vi "Read (Single Waveform).vi"(8 "error in (no error)":errorcluster, 9 "Maximum Time (10000ms)":u32=10000, 10 "Channel (0: Channel 1)":u16(ring) items=["Channel 1", "Channel 2", "Channel 3", "Channel 4", "Math", "Reference 1", "Reference 2", "Reference 3", "Reference 4", "D0", "D1", "D2", "D3", "D4", "D5", "D6", "D7", "D8", "D9", "D10", "D11", "D12", "D13", "D14", "D15", "Amplitude", "Frequency", "Phase", "Normal", "Average", "Maximum Peak Hold", "Minimum Peak Hold"], 11 "VISA resource name":refnum<visa-resource-name>) -> (0 "error out":errorcluster, 2 "Waveform Graph":waveform(dbl)(graph), 3 "VISA resource name out":refnum<visa-resource-name>)   [LabVIEW 2013, in "Tektronix DPO MSO 2000 4000 Series.lvlib"]
doc: "Initiates an acquisition on all channels that you enabled with the Configure Channel VI. This VI waits for the acquisition to complete and returns the waveform for the <B> Channel</B> you specify. The <B>Timeout</B> control specifies the maximum time to wait for operation complete in milliseconds. If the oscilloscope does not complete the acquisition within the time period you specify in <B>Timeout</B>, this VI returns a timeout error. A timeout error can occur when the trigger level is out of the range of the waveform.\n\nUse the tkdpo4k Fetch Waveform VI to obtain the waveforms for each of the remaining enabled <B>Source Channels</B> without initiating another acquisition.\n\nNote: If the instrument does not support auto-compensation for probe attenuation, adjust the scaling of the waveform data accordingly. You can adjust the scaling of the waveform data either automatically by using the tkdpo4k Configure Channel VI or manually by multiplying the waveform data by the probe attenuation."
uses:
  Tektronix DPO MSO 2000 4000 Series.lvlib
  Data_Low Level/Fetch Waveform (Waveform Data Type).vi
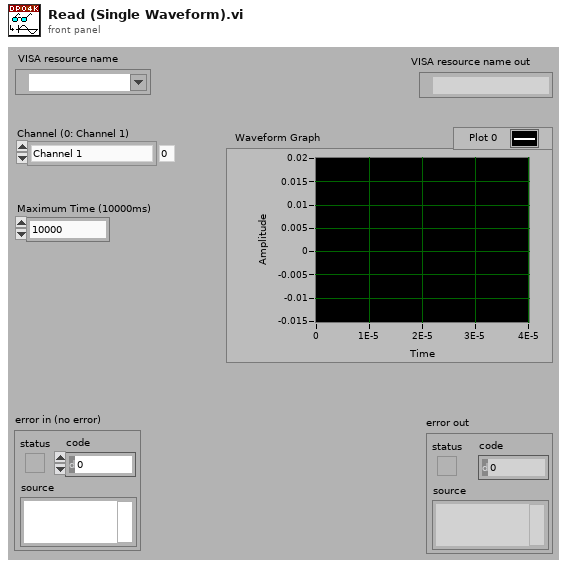
[diagram p1: front panel]
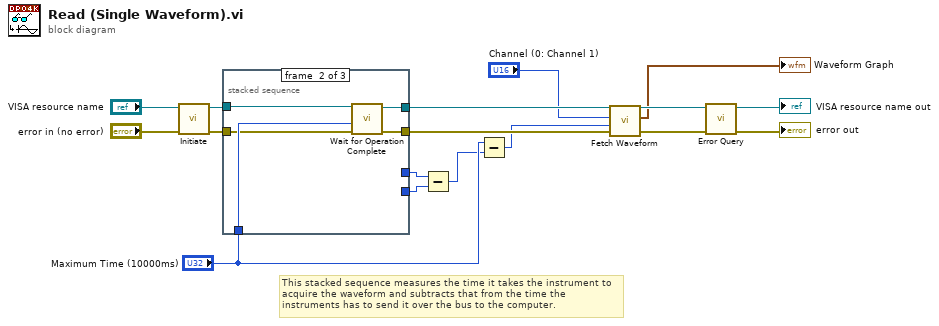
[diagram p0: block diagram]
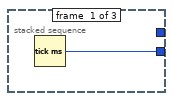
[diagram p2: hidden frame]
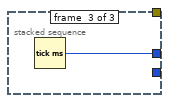
[diagram p3: hidden frame]
diagram:
  # "This stacked sequence measures the time it takes the instrument to acquire the waveform and subtracts that from the time the instruments has to send it over the bus to the computer."
  n1 = call "Initiate.vi"("error in (no error)"="error in (no error)", "VISA resource name"="VISA resource name") -> ("error out"=w12:errorcluster, "VISA resource name out"=w13:refnum<visa-resource-name>)  [unwired: 8 in]
  n2 = stacked-sequence {
    tunnel: w13 -> [_ w22 _]
    tunnel: w12 -> [_ w21 _]
    tunnel: "Maximum Time (10000ms)" -> [_ w23 _]
    tunnel: [_ w20 _] -> w11
    tunnel: [_ w19 _] -> w10
    tunnel: [_ _ w24] -> w7
    tunnel: [w18 _ _] -> w6
    frame #0 {
      n3 = Tick Count (ms)() -> (millisecond timer value=w18:u32)
    }
    frame #1 {
      n4 = call "Wait for Operation Complete.vi"("error in (no error)"=w21, "Maximum Time (10000ms)"=w23, "VISA resource name"=w22) -> ("error out"=w19:errorcluster, "VISA resource name out"=w20:refnum<visa-resource-name>)  [unwired: 7 in]
    }
    frame #2 {
      n5 = Tick Count (ms)() -> (millisecond timer value=w24:u32)
    }
  }
  n6 = Subtract(x=w7, y=w6) -> (x-y=w4:u32)
  n7 = Subtract(x="Maximum Time (10000ms)", y=w4) -> (x-y=w3:u32)
  n8 = call-poly "Fetch Waveform.vi"("error in (no error)"=w10, "Maximum Time (10000ms)"=w3, "Channel (0: Channel 1)"="Channel (0: Channel 1)", "VISA resource name"=w11) -> ("error out"=w8:errorcluster, "Waveform Data"=→"Waveform Graph":waveform(dbl), "VISA resource name out"=w9:refnum<visa-resource-name>)  [unwired: 5 in]
  n9 = call "Error Query.vi"("error in (no error)"=w8, "VISA resource name"=w9) -> ("error out"=→"error out":errorcluster, "VISA resource name out"=→"VISA resource name out":refnum<visa-resource-name>)  [unwired: 6 in, 2 out]
